vi "Update Number of Frames Done.vi"(8 "Increment?":bool, 9 "Reset":bool, 11 "Records Done":u32) -> (3 "Updated Records Done":u32)   [LabVIEW 2014]
panel:
  # "Copyright 2014 Vidrio Technologies\nScanImage 5 software is licensed under the Apache License, Version 2.0 (the \"License\"); you may not use any files contained\nwithin the ScanImage 5 release except in compliance with the License. You may obtain a copy of the License at\n http://www.apache.org/licenses/LICENSE-2.0\nUnless required by applicable law or agreed to in writing, software distributed under the License is distributed on an\n\"AS IS\" BASIS, WITHOUT WARRANTIES OR CONDITIONS OF ANY KIND, either express or implied. See the License for the\n specific language governing permissions and limitations under the License."
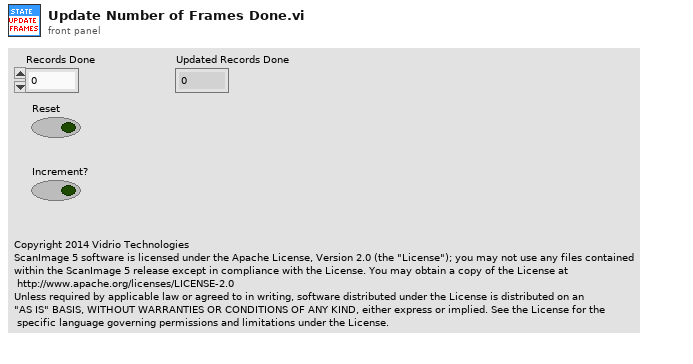
[diagram p1: front panel]
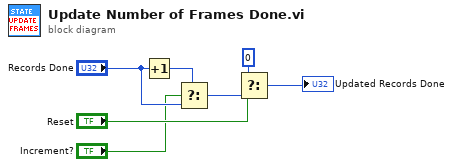
[diagram p0: block diagram]
diagram:
  n1 = Increment(x="Records Done") -> (x+1=w7:u32)
  n2 = Select(t=w7, s="Increment?", f="Records Done") -> (s? t:f=w6:u32)
  n3 = Select(t=u32 0, s="Reset", f=w6) -> (s? t:f=→"Updated Records Done":u32)
